vi "Add Active DUT SIM Slot.vi"(8 "error in (no error)":errorcluster, 10 "SIM Profile (\"SIMProfile\")":string="SIMProfile", 11 "VISA resource name":refnum<visa-resource-name>) -> (0 "error out":errorcluster, 3 "VISA resource name out":refnum<visa-resource-name>)   [LabVIEW 2020, in "Rohde&Schwarz CMXP Base.lvlib"]
doc: "Adds a SIM slot with the assigned SIM profile name to the active DUT.\n\nAssign a unique name to each named object within the test environment. Assigning an already used name can be rejected with an error message, even if the other object has not the same type as the new object.\n\nAttribute:\nRSCMXPBASE_ATTR_ACTIVE_DUT_SIM_SLOT_ADD\n\nRemote-control command:\nCREate:DUT:SIMSlot"
uses:
  <instrlib>/Rohde&Schwarz CMXP Base/Rohde&Schwarz CMXP Base.lvlib
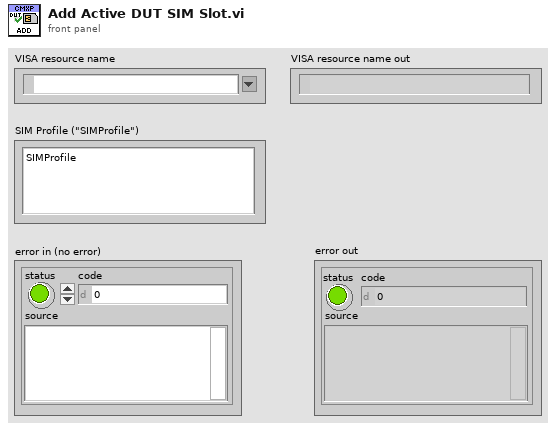
[diagram p1: front panel]
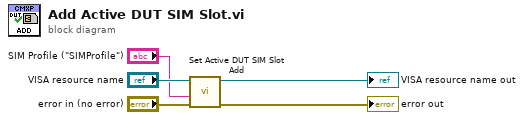
[diagram p0: block diagram]
diagram:
  n1 = call "Set Active DUT SIM Slot Add"("error in (no error)"="error in (no error)", "Active DUT SIM Slot Add ()"="SIM Profile (\"SIMProfile\")", "instrument handle"="VISA resource name") -> ("error out"=→"error out":errorcluster, "instrument handle out"=→"VISA resource name out":refnum<visa-resource-name>)  [unwired: 7 in]
